vi "myRIO_BRig_RT__Case_Exp_State_Reward.vi"(0 "input_dataCurrent":u16[](array[numeric]), 5 "input_state":T1, 9 "input_spout":enum16{"Left", "Right"}(ring)) -> (4 "output_dataCurrent":u16[](array[numeric]), 6 "output_state":T1, 8 "output__L":bool, 10 "output__R":bool)   [LabVIEW 2014]
uses:
  myRIO_BRig_RT__Case_Exp_stateList.ctl
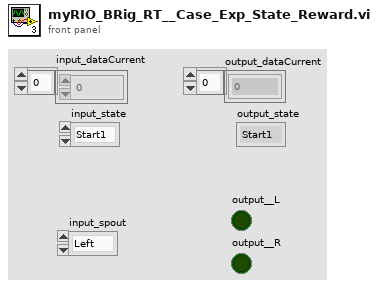
[diagram p1: front panel]
types:
  T1 = typedef "myRIO_BRig_RT__Case_Exp_stateList.ctl" = enum16{"Start1", "Start2", "Start3", "saveSettings1", "saveSettings2", "saveSettings3", "saveSettings4", "saveSettings_LC_ENL_l1", "saveSettings_LC_ENL_l2", "saveSettings_LC_Cue_l1", "saveSettings_LC_Cue_l2", "saveSettings6_LC_l1_Other", "SaveSettings6_LC_l2_Other", "setSettings_Audio", "setSettings_Laser", "initBlock_pre", "initBlock", "initBlock2", "initBlock_post", "initTrial_pre", "initTrial", "initTrial2", "initTrial3", "initTrial4", "initTrial_LC_ENL1", "initTrial_LC_Cue1", "initTrial_LC_Cue1_2", "initTrial_LC_Sel", "initTrial_post", "ENL1_pre", "ENL1", "ENL1_post", "ENL1Penalty_pre", "ENL1Penalty", "ENL2_pre", "ENL2", "ENL2Penalty_pre", "ENL2Penalty", "Cue1_pre", "Cue1", "Cue1_post", "Cue1Penalty_pre", "Cue1Penalty", "Cue2_pre", "Cue2", "Cue2Penalty_pre", "Cue2Penalty", "Selection_pre", "Selection", "Select_post", "SelectReward_pre", "SelectReward", "SelectRewardPost_pre", "SelectRewardPost", "SelectWrong_pre", "SelectWrong", "SelectWrong_post", "SelectTimeout_pre", "SelectTimeout", "SelectTimeout_post", "endTrial_pre", "endTrial1", "endTrial2", "endTrial3", "endTrial_post", "endBlock_pre", "endBlock", "endBlock_post", "endExp", "commConnect", "commUpload_pre", "commUpload_dataBlock", "commUpload_dataCurrent", "commUpload_dataExp", "commUpload_dataLC", "commUpload_dataTrial", "commUpload_post", "saveData_pre", "saveData_dataBlock", "saveData_dataCurrent", "saveData_dataExp", "saveData_dataLC", "saveData_dataTrial", "saveData_post", "empty_endBlock1", "empty_endBlock2", "empty_endTrial1", "empty_endTrial2", "empty_endTrial3", "empty_endTrial4", "empty_endTrial5", "dummyState", "dummyState_endBlock"}
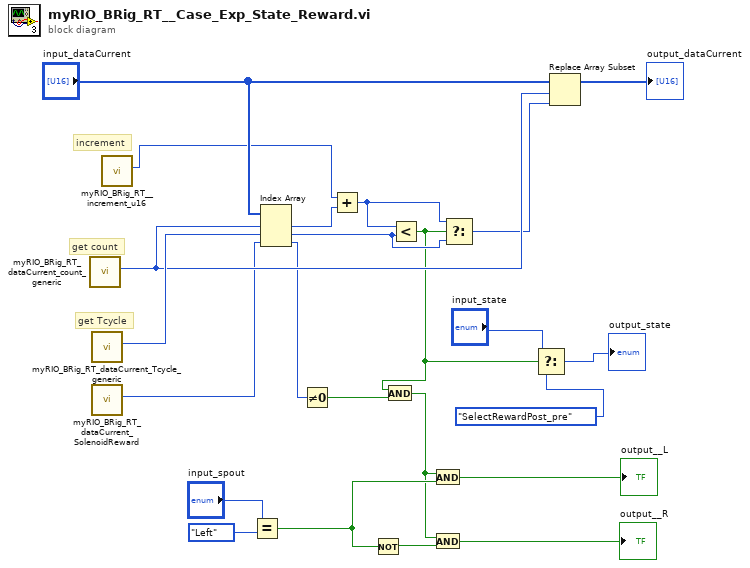
[diagram p0: block diagram]
diagram:
  # "increment"
  # "get Tcycle"
  # "get count"
  n1 = call "myRIO_BRig_RT_dataCurrent_count_generic.vi"() -> ("output_count_generic"=w19:i32)  [unwired: 11 in]
  n2 = call "myRIO_BRig_RT_dataCurrent_Tcycle_generic.vi"() -> ("output_Tcycle_generic"=w21:i32)  [unwired: 11 in]
  n3 = call "myRIO_BRig_RT_dataCurrent_SolenoidReward.vi"() -> ("output_SolenoidReward"=w6:i32)  [unwired: 11 in]
  n4 = call "myRIO_BRig_RT__increment_u16.vi"() -> ("output_increment__u16"=w11:u16)  [unwired: 11 in]
  n5 = Equal?(x="input_spout", y=enum16{"Left", "Right"}."Left") -> (x = y?=w12:bool)
  n6 = Index Array(array="input_dataCurrent", index #1=w19, index #2=w21, index #3=w6) -> (element #1=w20:u16, element #2=w18:u16, element #3=w5:u16)
  n7 = Not Equal To 0?(x=w5) -> (x != 0?=w3:bool)
  n8 = Add(x=w11, y=w20) -> (x+y=w10:u16)
  n9 = Not(x=w12) -> (.not. x?=w14:bool)
  n10 = Less?(x=w10, y=w18) -> (x < y?=w2:bool)
  n11 = And(x=w2, y=w3) -> (x .and. y?=w1:bool)
  n12 = And(x=w1, y=w12) -> (x .and. y?=→"output__L":bool)
  n13 = And(x=w1, y=w14) -> (x .and. y?=→"output__R":bool)
  n14 = Select(t=w10, s=w2, f=w18) -> (s? t:f=w17:u16)
  n15 = Select(t="input_state", s=w2, f=myRIO_BRig_RT__Case_Exp_stateList."SelectRewardPost_pre" ("Enum")) -> (s? t:f=→"output_state":T1)
  n16 = Replace Array Subset(array="input_dataCurrent", new element=w17, index=w19) -> (→"output_dataCurrent":u16[])
